vi "Clear Fault.vi"(8 "error in (no error)":errorcluster, 10 "fault code":i32, 11 "target address (localhost)":string="localhost") -> (0 "error out":errorcluster)   [LabVIEW 2020]
doc: "Clears NI Scan Engine faults. If the fault you specify using the <B>fault code</B> input is active, this VI clears the fault. If the fault is not active, this VI takes no action and generates no error."
uses:
  <resource>/objmgr/ni.var.rc
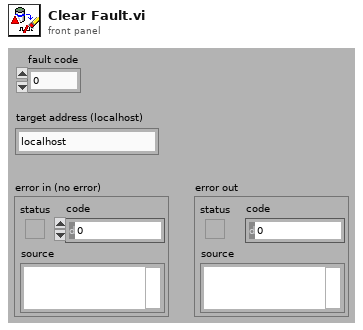
[diagram p1: front panel]
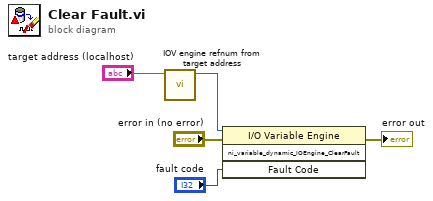
[diagram p0: block diagram]
diagram:
  n1 = call <vilib>:"IOV engine refnum from target address.vi"("target address"="target address (localhost)") -> ("reference out"=w4:refnum<k21>)  [unwired: 10 in]
  n2 = invoke class="I/O Variable Engine" method="ni_variable_dynamic_IOEngine_ClearFault"(reference=w4, error in="error in (no error)", "Fault Code"="fault code") -> (error out=→"error out":errorcluster)  [unwired: 1 in, 3 out]
